vi "Auton - Center Gear-Baseline.vi"(10 "Baseline Direction":enum16{"Right", "Left"}(ring), 11 "Auton States":T1=enum."Reset Encoders") -> ()   [LabVIEW 2016]
uses:
  Auton - Center Gear-Basline States.ctl
panel:
  in  "Cross Baseline SP":dbl
  in  "Turn Right SP":dbl
  in  "Turn Left SP":dbl
  in  "Back Away SP":dbl
  in  "Drive Forward SP":dbl=90.0
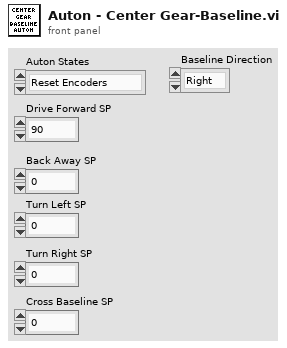
[diagram p1: front panel]
types:
  T1 = typedef "Auton - Center Gear-Basline States.ctl" = enum16{"Stop", "Reset Encoders", "Drive Forward", "Eject Gear", "Back Away", "Turn Away from Airship", "Reset Encoders Again", "Cross Baseline"}
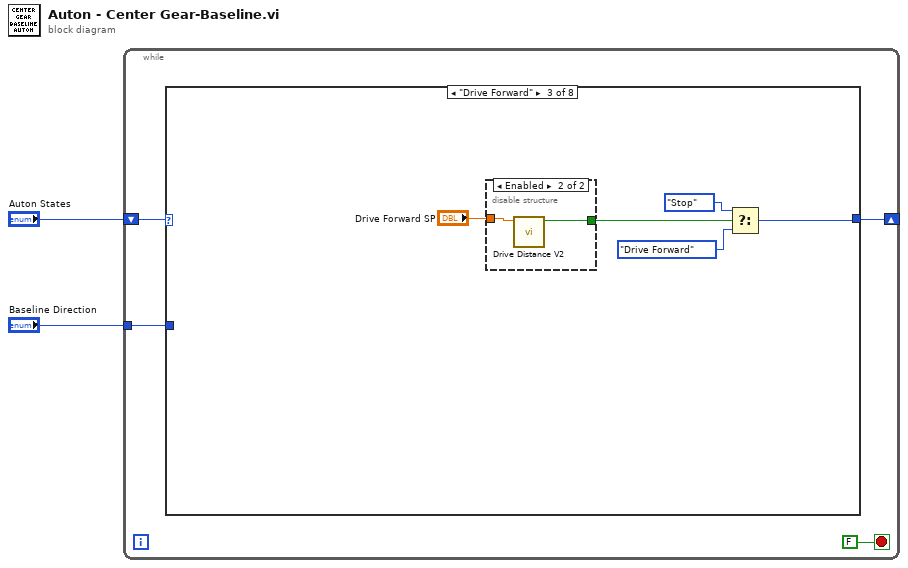
[diagram p0: block diagram]
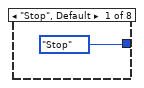
[diagram p2: hidden frame]
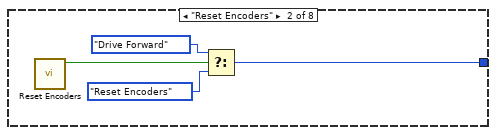
[diagram p3: hidden frame]
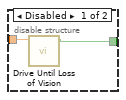
[diagram p4: hidden frame]
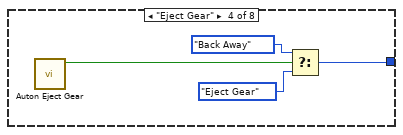
[diagram p5: hidden frame]
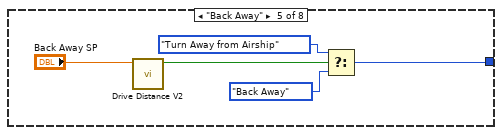
[diagram p6: hidden frame]
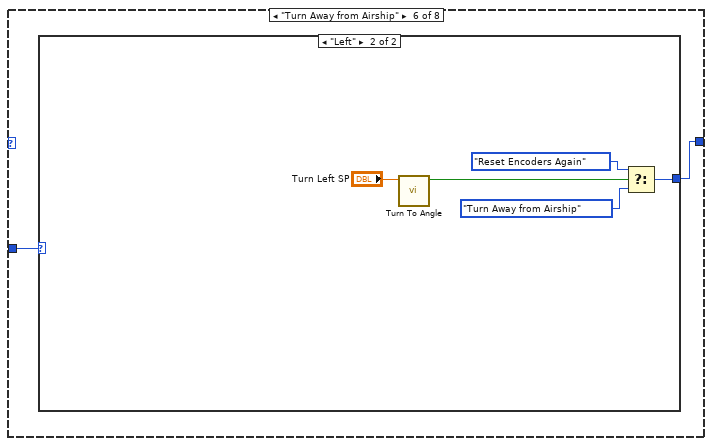
[diagram p7: hidden frame]
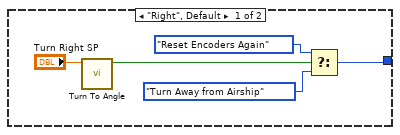
[diagram p8: hidden frame]
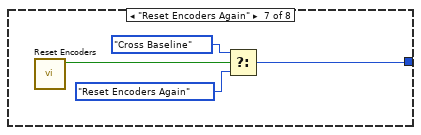
[diagram p9: hidden frame]
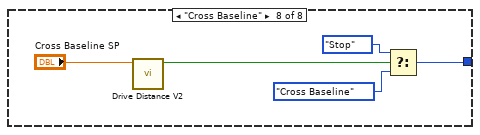
[diagram p10: hidden frame]
diagram:
  n1 = while {
    shift-right: [w5] -> _
    shift-left: "Auton States" -> [w6]
    tunnel: "Baseline Direction" -> [w4]
    stop <- FALSE stop-if-true
    n2 = case shown="\"Drive Forward\"" w6 {
      tunnel: [Auton_-_Center_Gear-Basline_States."Stop" ("Auton States 2") w8 w14 w22 w27 w30 w42 w48] -> w5
      tunnel: w4 -> [_ _ _ _ _ w31 _ _]
      frame "Stop", Default {
      }
      frame "Reset Encoders" {
        n3 = call "Reset Encoders.vi"() -> ("Done?"=w10:bool)  [unwired: 11 in]
        n4 = Select(t=Auton_-_Center_Gear-Basline_States."Drive Forward" ("Auton States 2"), s=w10, f=Auton_-_Center_Gear-Basline_States."Reset Encoders" ("Auton States 2")) -> (s? t:f=w8:T1)
      }
      frame "Drive Forward" {
        n5 = disable-structure shown="Enabled" {
          disable-tunnel: "Drive Forward SP" -> [w18 w20]
          disable-tunnel: [w17 w19] -> w12
          frame Disabled {
            n6 = call "Drive Until Loss of Vision.vi"("Distance SP"=w18) -> ("Lost Vision (ready to approach)"=w17:bool)  [unwired: 10 in]
          }
          frame Enabled {
            n7 = call "Drive Distance V2.vi"("Distance Set Point"=w20) -> ("Done?"=w19:bool)  [unwired: 10 in]
          }
        }
        n8 = Select(t=Auton_-_Center_Gear-Basline_States."Stop" ("Auton States 2"), s=w12, f=Auton_-_Center_Gear-Basline_States."Drive Forward" ("Auton States 2")) -> (s? t:f=w14:T1)
      }
      frame "Eject Gear" {
        n9 = call "Auton Eject Gear.vi"() -> ("Done?"=w21:bool)  [unwired: 11 in]
        n10 = Select(t=Auton_-_Center_Gear-Basline_States."Back Away" ("Auton States 2"), s=w21, f=Auton_-_Center_Gear-Basline_States."Eject Gear" ("Auton States 2")) -> (s? t:f=w22:T1)
      }
      frame "Back Away" {
        n11 = call "Drive Distance V2.vi"("Distance Set Point"="Back Away SP") -> ("Done?"=w26:bool)  [unwired: 10 in]
        n12 = Select(t=Auton_-_Center_Gear-Basline_States."Turn Away from Airship" ("Auton States 2"), s=w26, f=Auton_-_Center_Gear-Basline_States."Back Away" ("Auton States 2")) -> (s? t:f=w27:T1)
      }
      frame "Turn Away from Airship" {
        n13 = case shown="\"Left\"" w31 {
          tunnel: [w32 w39] -> w30
          frame "Right", Default {
            n14 = call "Turn To Angle.vi"("Setpoint"="Turn Right SP") -> ("Done?"=w35:bool)  [unwired: 10 in]
            n15 = Select(t=Auton_-_Center_Gear-Basline_States."Reset Encoders Again" ("Auton States 2"), s=w35, f=Auton_-_Center_Gear-Basline_States."Turn Away from Airship" ("Auton States 2")) -> (s? t:f=w32:T1)
          }
          frame "Left" {
            n16 = call "Turn To Angle.vi"("Setpoint"="Turn Left SP") -> ("Done?"=w38:bool)  [unwired: 10 in]
            n17 = Select(t=Auton_-_Center_Gear-Basline_States."Reset Encoders Again" ("Auton States 2"), s=w38, f=Auton_-_Center_Gear-Basline_States."Turn Away from Airship" ("Auton States 2")) -> (s? t:f=w39:T1)
          }
        }
      }
      frame "Reset Encoders Again" {
        n18 = call "Reset Encoders.vi"() -> ("Done?"=w44:bool)  [unwired: 11 in]
        n19 = Select(t=Auton_-_Center_Gear-Basline_States."Cross Baseline" ("Auton States 2"), s=w44, f=Auton_-_Center_Gear-Basline_States."Reset Encoders Again" ("Auton States 2")) -> (s? t:f=w42:T1)
      }
      frame "Cross Baseline" {
        n20 = call "Drive Distance V2.vi"("Distance Set Point"="Cross Baseline SP") -> ("Done?"=w47:bool)  [unwired: 10 in]
        n21 = Select(t=Auton_-_Center_Gear-Basline_States."Stop" ("Auton States 2"), s=w47, f=Auton_-_Center_Gear-Basline_States."Cross Baseline" ("Auton States 2")) -> (s? t:f=w48:T1)
      }
    }
  }
